vi "spot size 2D.vi"(6 "ImageSum":ext, 8 "error in (no error)":errorcluster, 9 "X Centroid":sgl, 10 "Y Centroid":sgl, 11 "Refnum in":T1) -> (0 "w0y via 2nd mom":sgl, 1 "w0x via 2nd mom":sgl, 2 "FWHMx (pix)":dbl, 3 "FWHMy (pix)":dbl, 4 "error out":errorcluster)   [LabVIEW 2020]
uses:
  IMAQ Image.ctl
  NI_Vision_Development_Module.lvlib
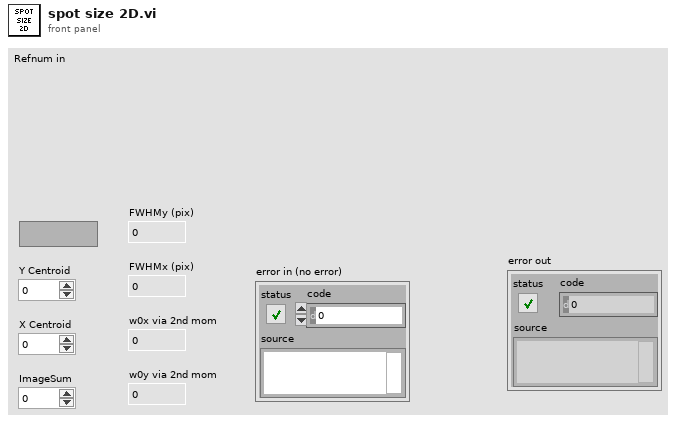
[diagram p1: front panel]
types:
  T1 = typedef "IMAQ Image.ctl" = refnum<image>
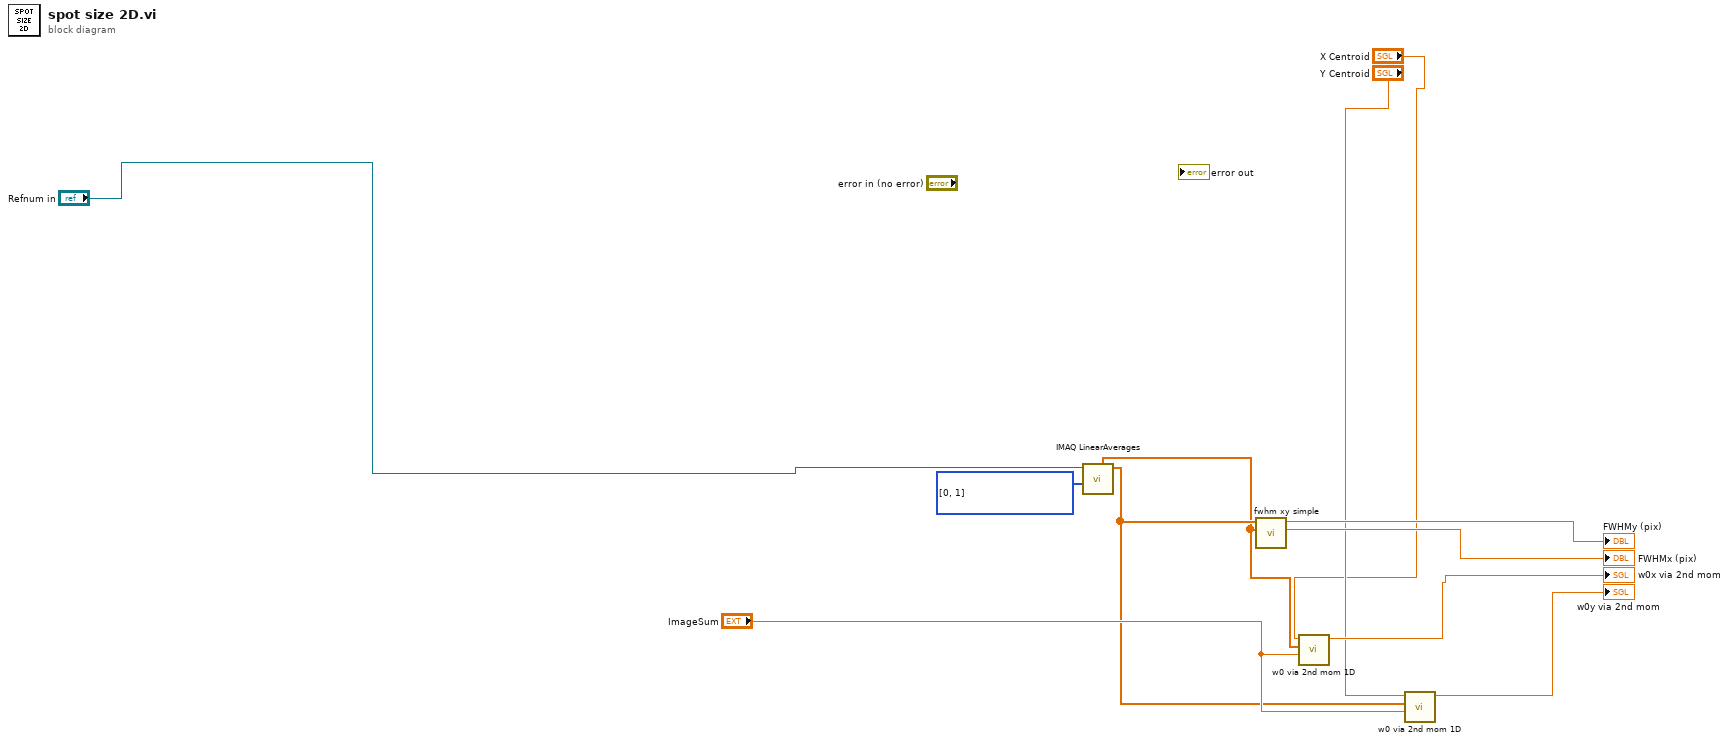
[diagram p0: block diagram]
diagram:
  w3 = i32[] [0, 1] items=["X Axis Averages", "Y Axis Averages", "X + Y Axis Averages", "X - Y Axis Averages"] ("Averages")
  n1 = call "IMAQ LinearAverages"("Averages"=w3, "Image Src"="Refnum in") -> ("Y Axis Averages"=w5:sgl[], "X Axis Averages"=w4:sgl[])  [unwired: 2 in, 6 out]
  n2 = call "fwhm xy simple.vi"("X Axis Averages"=w4, "Y Axis Averages"=w5) -> ("FWHM (pix) 2"=→"FWHMx (pix)":dbl, "FWHM (pix)"=→"FWHMy (pix)":dbl)  [unwired: 8 in]
  n3 = call "w0 via 2nd mom 1D.vi"("Sum"="ImageSum", "Input array"=w4, "Centroid"="X Centroid") -> ("w0 via 2nd mom"=→"w0x via 2nd mom":sgl)  [unwired: 8 in]
  n4 = call "w0 via 2nd mom 1D.vi"("Sum"="ImageSum", "Input array"=w5, "Centroid"="Y Centroid") -> ("w0 via 2nd mom"=→"w0y via 2nd mom":sgl)  [unwired: 8 in]
